vi "CMN_Read_Lines_From_File.vi"(2 "convert eol? (no:F)":bool, 3 "file path":path, 4 "number of lines (all:-1)":i32=-1, 8 "start of read offset (chars.:0)":i32, 9 "[max characters per line]  (no limit:0)":i32) -> (0 "new file path (Not A Path if cancelled)":path, 1 "line string":string, 5 "mark after read (chars.)":i32, 6 "EOF?":bool)   [LabVIEW 2016]
doc: "LabVIEW no longer supports this VI. Use the Read Text function instead. Reads a specified number of lines from a byte stream file beginning at a specified character offset. The VI opens the file before reading from it and closes it afterwards."
panel:
  in  "prompt":string="Choose file to read."
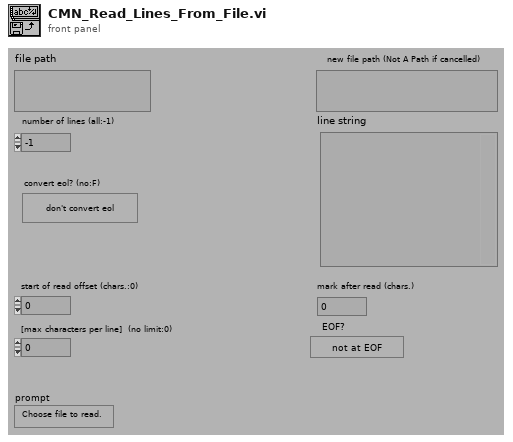
[diagram p1: front panel]
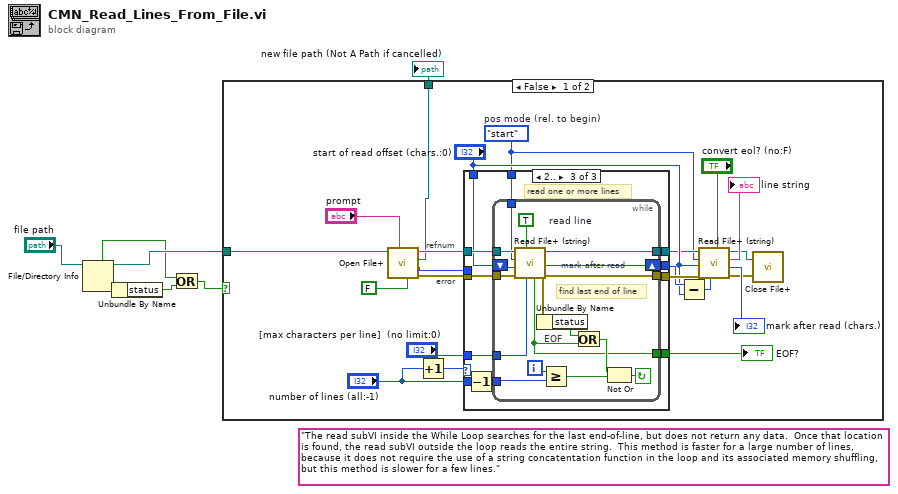
[diagram p0: block diagram]
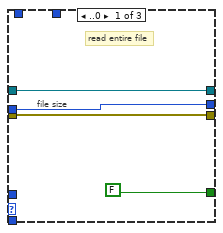
[diagram p2: hidden frame]
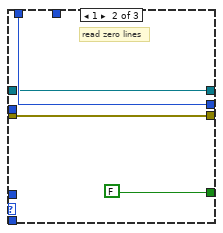
[diagram p3: hidden frame]
diagram:
  (unwired) "The read subVI inside the While Loop searches for the last end-of-line, but does not return any data.  Once that location is found, the read subVI outside the loop reads the entire string.  This method is faster for a large number of lines, because it does not require the use of a string concatentation function in the loop and its associated memory shuffling, but this method is slower for a few lines."
  n1 = File/Directory Info(path="file path") -> (path out=w7:path, directory=w2:bool, error out=w4:errorcluster)  [unwired: 1 in, 4 out]
  n2 = Unbundle By Name(w4) -> ("status"=w3:bool)
  n3 = Or(x=w2, y=w3) -> (x .or. y?=w1:bool)
  n4 = case shown="False" w1 {
    tunnel: w7 -> [w12 w65]
    tunnel: [w9 w65] -> w6
    frame False {
      w17 = enum16{"start", "end", "current"}."start"  # pos mode (rel. to begin)
      # "error"
      # "refnum"
      n5 = call <vilib>:"Open File+.vi"("advisory dialog? (display:T)"=FALSE, "prompt"="prompt", "file path (\" \")"=w12) -> ("error out"=w16:errorcluster, "file size (bytes)"=w15:i32, "file path"=w9:path, "refnum"=w14:refnum<file>)  [unwired: 4 in, 1 out]
      n6 = Increment(x="number of lines (all:-1)") -> (x+1=w23:i32)
      n7 = case shown="2.." w23 {
        tunnel: [w33 w36 w48] -> w25
        tunnel: [w32 w37 w47] -> w24
        tunnel: "number of lines (all:-1)" -> [_ _ w46]
        tunnel: "[max characters per line]  (no limit:0)" -> [_ _ w45]
        tunnel: w16 -> [w33 w36 w44]
        tunnel: w14 -> [w31 w35 w43]
        tunnel: "start of read offset (chars.:0)" -> [_ w37 w42]
        tunnel: w17 -> [_ _ w41]
        tunnel: w15 -> [w32 _ _]
        tunnel: [w31 w35 w40] -> w20
        tunnel: [FALSE FALSE w39] -> w19
        frame ..0 {
          # "file size"
          # "read entire file"
        }
        frame 1 {
          # "read zero lines"
        }
        frame 2.. {
          # "read one or more lines"
          n8 = Decrement(x=w46) -> (x-1=w38:i32)
          n9 = while {
            tunnel: [w50] -> w39
            tunnel: w41 -> [w55]
            tunnel: w44 -> [w57]
            tunnel: w45 -> [w58]
            tunnel: [w53] -> w48
            tunnel: w43 -> [w60]
            tunnel: [w61] -> w40
            tunnel: w38 -> [w49]
            shift-left: w42 -> [w62]
            shift-right: [w64] -> w47
            i -> [w63]
            stop <- w56 continue-if-true
            w52 = TRUE  # read line
            # "mark after read"
            # "find last end of line"
            # "EOF"
            n10 = call <vilib>:"Read File+ (string).vi"("count"=w58, "line mode (characters:F)"=w52, "error in (no error)"=w57, "pos offset (bytes:0)"=w62, "pos mode (rel. to current:2)"=w55, "refnum"=w60) -> ("error out"=w53:errorcluster, "mark after read (bytes)"=w64:i32, "dup refnum"=w61:refnum<file>, "EOF?"=w50:bool)  [unwired: 2 out]
            n11 = Unbundle By Name(w53) -> ("status"=w51:bool)
            n12 = Greater Or Equal?(x=w63, y=w49) -> (x >= y?=w59:bool)
            n13 = Or(x=w51, y=w50) -> (x .or. y?=w54:bool)
            n14 = Not Or(1:w59, 2:w54) -> (0:w56:bool)
          }
        }
      }
      "EOF?" <- w19
      n15 = Subtract(x=w24, y="start of read offset (chars.:0)") -> (x-y=w29:i32)
      n16 = call <vilib>:"Read File+ (string).vi"("convert eol? (no:F)"="convert eol? (no:F)", "count"=w29, "error in (no error)"=w25, "pos offset (bytes:0)"="start of read offset (chars.:0)", "pos mode (rel. to current:2)"=w17, "refnum"=w20) -> ("error out"=w11:errorcluster, "mark after read (bytes)"=→"mark after read (chars.)":i32, "string"=→"line string":string, "dup refnum"=w10:refnum<file>)  [unwired: 2 out]
      n17 = call <vilib>:"Close File+.vi"("error in (no error)"=w11, "refnum"=w10) -> ()  [unwired: 6 out]
    }
    frame True {
    }
  }
  "new file path (Not A Path if cancelled)" <- w6
